vi "增加用户.vi"(6 "用户名in":string[](array[string]), 10 "权限in":i32=2 min=2 max=3 step=1) -> (1 "取消":bool, 2 "用户信息":string[](array[string]))   [LabVIEW 2020]
panel:
  in  "确认密码":string
  in  "Btn_Exit":bool
  in  "Btn_Confirm":bool
  in  "权限":u16(ring) items=["操作员"]
  in  "密码":string
  in  "用户名":string
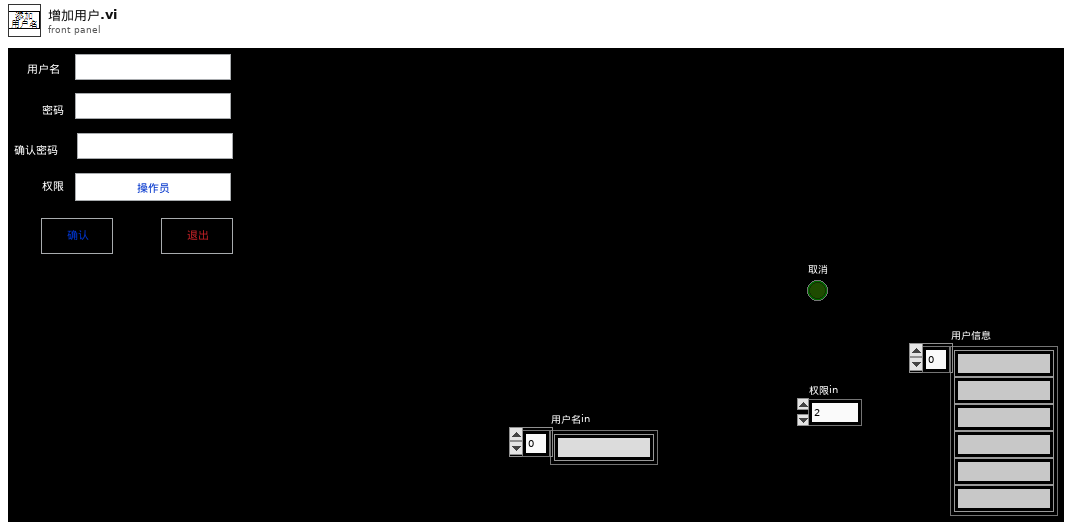
[diagram p1: front panel]
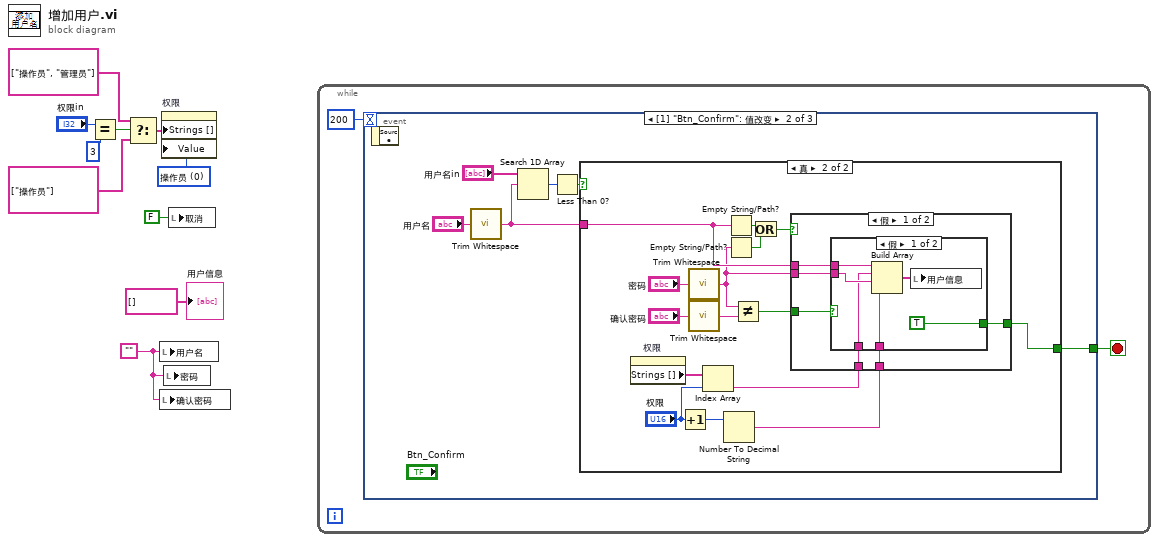
[diagram p0: block diagram]
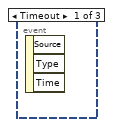
[diagram p2: hidden frame]
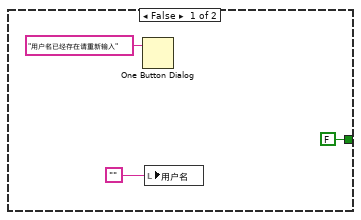
[diagram p3: hidden frame]
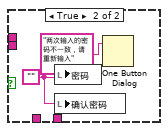
[diagram p4: hidden frame]
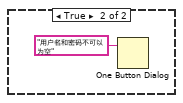
[diagram p5: hidden frame]
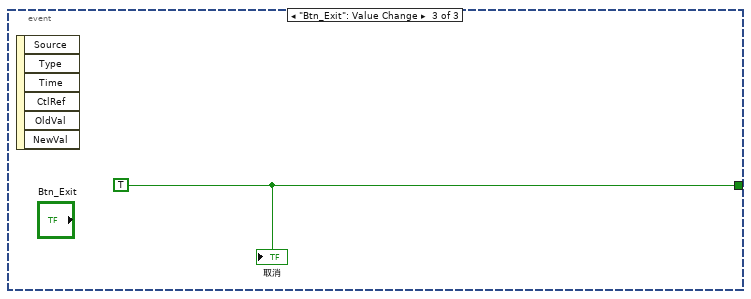
[diagram p6: hidden frame]
diagram:
  w1 = u16 0 items=["操作员"] ("权限")
  w2 = "" ("用户名")
  n1 = Equal?(x="权限in", y=3) -> (x = y?=w8:bool)
  n2 = Select(t=string[] ["操作员", "管理员"], s=w8, f=string[] ["操作员"]) -> (s? t:f=w5:string[])
  n3 = local write "用户名"(w2) -> ()
  n4 = local write "确认密码"(w2) -> ()
  n5 = property on="权限" class="Ring (严格)"("Strings []"=w5, "Value"=w1) -> ()  [unwired: 2 in, 2 out]
  n6 = local write "密码"(w2) -> ()
  n7 = local write "取消"(FALSE ("取消")) -> ()
  n8 = while {
    stop <- w11 stop-if-true
    n9 = event shown="[1] \"Btn_Confirm\": 值改变" {
      selector: _ -> [_ _ _]
      dyn-events: _ -> [_ _ _]
      timeout: 200 -> [_ _ _]
      tunnel: [_ w18 w52] -> w11
      event Timeout {
        n10 = event-data() -> ()  [unwired: 1 in, 3 out]
      }
      event "Btn_Confirm": Value Change {
        n11 = event-data() -> ()  [unwired: 1 in, 1 out]
        n12 = call <vilib>:"Trim Whitespace.vi"("string"="用户名") -> ("trimmed string"=w13:string)  [unwired: 1 in]
        n13 = Search 1D Array(1D array="用户名in", element=w13) -> (index of element=w15:i32)  [unwired: 1 in]
        n14 = Less Than 0?(x=w15) -> (x < 0?=w14:bool)
        n15 = case shown="真" w14 {
          tunnel: [FALSE w25] -> w18
          tunnel: w13 -> [_ w24]
          frame False {
            n16 = One Button Dialog(message="用户名已经存在请重新输入" ("消息")) -> ()  [unwired: 1 in, 1 out]
            n17 = local write "用户名"("" ("用户名")) -> ()
          }
          frame True {
            n18 = property on="权限" class="Ring (严格)"() -> ("Strings []"=w36:string[])  [unwired: 2 in, 2 out]
            n19 = Increment(x="权限") -> (x+1=w33:u16)
            n20 = call <vilib>:"Trim Whitespace.vi"("string"="密码") -> ("trimmed string"=w23:string)  [unwired: 1 in]
            n21 = call <vilib>:"Trim Whitespace.vi"("string"="确认密码") -> ("trimmed string"=w22:string)  [unwired: 1 in]
            n22 = Index Array(array=w36, index="权限") -> (element=w34:string)
            n23 = Number To Decimal String(number=w33) -> (decimal integer string=w32:string)  [unwired: 1 in]
            n24 = Empty String/Path?(string/path=w24) -> (empty?=w31:bool)
            n25 = Empty String/Path?(string/path=w23) -> (empty?=w30:bool)
            n26 = Not Equal?(x=w23, y=w22) -> (x != y?=w26:bool)
            n27 = Or(x=w31, y=w30) -> (x .or. y?=w29:bool)
            n28 = case shown="假" w29 {
              tunnel: w34 -> [w42 _]
              tunnel: w32 -> [w41 _]
              tunnel: w24 -> [w40 _]
              tunnel: w23 -> [w39 _]
              tunnel: w26 -> [w38 _]
              tunnel: [w37 _] -> w25
              frame False {
                n29 = case shown="假" w38 {
                  tunnel: w42 -> [w43 _]
                  tunnel: w41 -> [w48 _]
                  tunnel: w40 -> [w46 _]
                  tunnel: w39 -> [w44 _]
                  tunnel: [TRUE _] -> w37
                  frame False {
                    n30 = Build Array(w46, w43, w44, w48) -> (w47:string[])
                    n31 = local write "用户信息"(w47) -> ()
                  }
                  frame True {
                    w49 = ""
                    n32 = local write "密码"(w49) -> ()
                    n33 = local write "确认密码"(w49) -> ()
                    n34 = One Button Dialog(message="两次输入的密码不一致，请重新输入" ("消息")) -> ()  [unwired: 1 in, 1 out]
                  }
                }
              }
              frame True {
                n35 = One Button Dialog(message="用户名和密码不可以为空" ("消息")) -> ()  [unwired: 1 in, 1 out]
              }
            }
          }
        }
      }
      event "Btn_Exit": Value Change {
        w52 = TRUE ("取消")
        n36 = event-data() -> ()  [unwired: 1 in, 6 out]
        "取消" <- w52
      }
    }
  }
  "用户信息" <- string[] [] ("用户信息")
